vi "sample3(SyncW).vi"() -> ()   [LabVIEW 2011]
panel:
  out "data out":cluster{"ID":u8, "Error":u16, "Data":u8[]}[](array[cluster]) {"Error" format="%04x"}
  in  "id3":u8=3 max=253
  in  "id2":u8=2 max=253
  in  "id1":u8=1 max=253
  in  "pos3":u16(knob) scale=0.0..4095.0
  in  "STOP":bool
  in  "pos2":u16(knob) scale=0.0..4095.0
  in  "pos1":u16(knob) scale=0.0..4095.0
  in  "COM":refnum<visa-resource-name> caption="COMポート"
  in  "Baudrate":i32=1000000
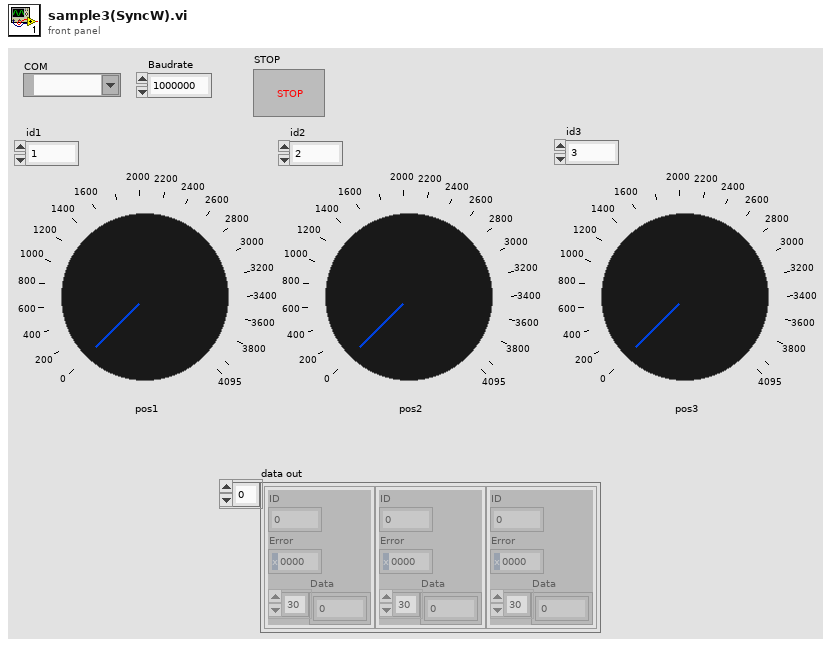
[diagram p1: front panel]
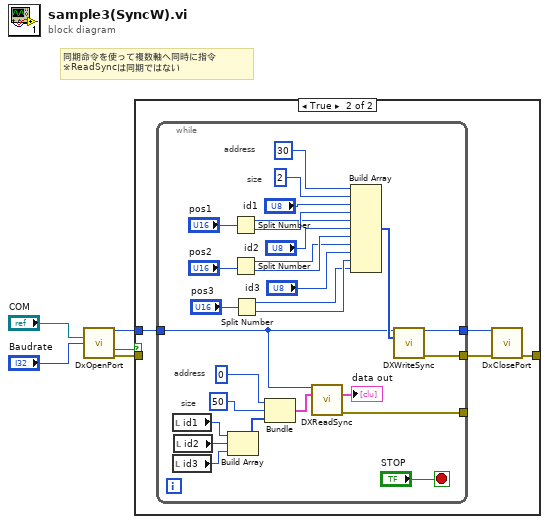
[diagram p0: block diagram]
diagram:
  # "同期命令を使って複数軸へ同時に指令\n※ReadSyncは同期ではない"
  n1 = call "DxOpenPort.vi"("port"="COM", "baudrate"="Baudrate") -> ("dvid"=w5:u32, "成功"=w2:bool, "エラー出力"=w1:errorcluster)  [unwired: 11 in]
  n2 = case shown="TRUE" w2 {
    tunnel: w5 -> [_ w10]
    tunnel: w1 -> [w6 _]
    tunnel: [w6 w7] -> _
    frame False {
    }
    frame True {
      n3 = while {
        tunnel: w10 -> [w20]
        tunnel: [w29] -> w9
        tunnel: [w27] -> w8
        tunnel: [w17] -> _
        stop <- "STOP" stop-if-true
        # "size"
        # "address"
        # "size"
        # "address"
        n4 = local read "id1"() -> (w19:u8)
        n5 = local read "id3"() -> (w11:u8)
        n6 = local read "id2"() -> (w18:u8)
        n7 = Build Array(w19, w18, w11) -> (w15:u8[])
        n8 = Split Number(x="pos1") -> (hi(x)=w31:u8, lo(x)=w32:u8)
        n9 = Split Number(x="pos2") -> (hi(x)=w33:u8, lo(x)=w34:u8)
        n10 = Split Number(x="pos3") -> (hi(x)=w25:u8, lo(x)=w26:u8)
        n11 = Bundle("OffsetAddr"=u8 0, "OffsetAddr"=u8 50, w15) -> (w12:cluster{"OffsetAddr":u8, "OffsetAddr":u8, u8[]})  [unwired: 1 in]
        n12 = call "DXReadSync.vi"("dvid in"=w20, "Param"=w12) -> ("data out"=→"data out":cluster{"ID":u8, "Error":u16, "Data":u8[]}[], "エラー出力"=w17:errorcluster)  [unwired: 10 in, 2 out]
        n13 = Build Array(u8 30 ("OffsetAddr"), u8 2 ("OffsetAddr"), "id1", w32, w31, "id2", w34, w33, "id3", w26, w25) -> (w35:u8[])
        n14 = call "DXWriteSync.vi"("dvid in"=w20, "data in"=w35) -> ("dvid out"=w27:u32, "エラー出力"=w29:errorcluster)  [unwired: 11 in, 1 out]
      }
      n15 = call "DxClosePort.vi"("dvid"=w8, "エラー入力"=w9) -> ("エラー出力"=w7:errorcluster)  [unwired: 12 in, 1 out]
    }
  }
